vi "Drive_Initialize.vi"(11 "HW SETUP_WC Drive":T1={"Left Master"=3, "Invert Left Master"=FALSE, "Left Slave"=6, "Invert Left Slave"=FALSE, "Right Master"=12, "Invert Right Master"=FALSE, "Right Slave"=13, "Invert Right Slave"=FALSE, "Invert Left Encoder"=TRUE, "Invert Right Encoder"=FALSE}) -> (3 "RobotDriveDevRef Out":T2)   [LabVIEW 2017, in "WCDrive2018.lvlib"]
uses:
  WCDrive2018.lvlib
  <vilib>/Rock Robotics/WPI/RobotDrive/WPI_RobotDriveDevRef.ctl
  <vilib>/Rock Robotics/WPI/MotorControl/WPI_MotorControlDeviceRef.ctl
  <vilib>/Rock Robotics/WPI/MotorControl/WPI_MotorControlType.ctl
  <vilib>/Rock Robotics/SystemInterfaces/DIO/FPGA_DIOPWMChannel.ctl
  <vilib>/Rock Robotics/WPI/PWM/WPI_PWMDeadband.ctl
  <vilib>/Rock Robotics/SystemInterfaces/DIO/FPGA_DIOChannel.ctl
  ProtoType Code/Claw Testing/Systems/WCDrive2018/Cluster_WCDrive_SetupData.ctl
  System Drivers/Phoenix-LabVIEW/Motor Controller/Controls/CTRE_Phoenix_MotorControl_FeedbackDevice.ctl
  System Drivers/Phoenix-LabVIEW/Motor Controller/Controls/CTRE_Phoenix_MotorControl_NeutralMode.ctl
  <vilib>/Rock Robotics/WPI/RobotDrive/WPI_RobotDriveOpen4MotorWithExistingMotors.vi
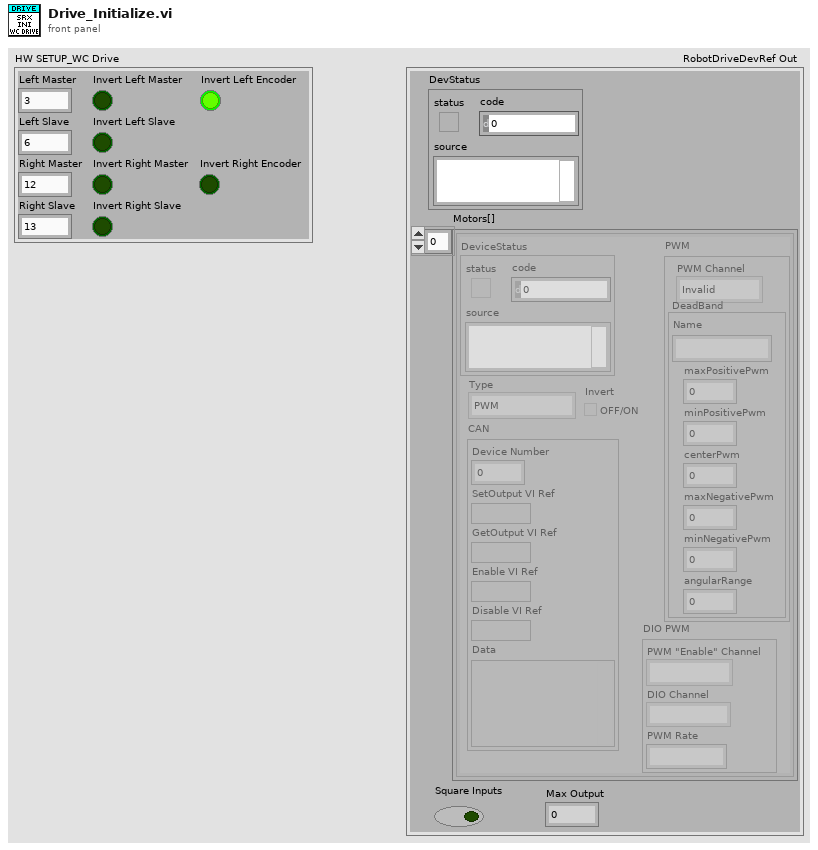
[diagram p1: front panel]
types:
  T1 = typedef "Cluster_WCDrive_SetupData.ctl" = cluster{"Left Master":u8, "Invert Left Master":bool, "Left Slave":u8, "Invert Left Slave":bool, "Right Master":u8, "Invert Right Master":bool, "Right Slave":u8, "Invert Right Slave":bool, "Invert Left Encoder":bool, "Invert Right Encoder":bool}
  T2 = typedef "WPI_RobotDriveDevRef.ctl" = cluster{"DevStatus":errorcluster, "Motors[]":T3[], "Square Inputs":bool, "Max Output":dbl}
  T3 = typedef "WPI_MotorControlDeviceRef.ctl" = cluster{"DeviceStatus":errorcluster, "Type":T4, "PWM":cluster{"PWM Channel":T5, "DeadBand":T6}, "CAN":cluster{"Device Number":u8, "SetOutput VI Ref":variant, "GetOutput VI Ref":variant, "Enable VI Ref":variant, "Disable VI Ref":variant, "Data":variant}, "Invert":bool, "DIO PWM":cluster{"PWM \"Enable\" Channel":T5, "DIOChannel":T7, "PWM Rate":dbl}}
  T4 = typedef "WPI_MotorControlType.ctl" = enum16{"PWM", "CAN", "DIO PWM"}
  T5 = typedef "FPGA_DIOPWMChannel.ctl" = enum8{"PWM 0", "PWM 1", "PWM 2", "PWM 3", "PWM 4", "PWM 5", "PWM 6", "PWM 7", "PWM 8", "PWM 9", "PWM MXP 0", "PWM MXP 1", "PWM MXP 2", "PWM MXP 3", "PWM MXP 4", "PWM MXP 5", "PWM MXP 6", "PWM MXP 7", "PWM MXP 8", "PWM MXP 9", "Invalid"}
  T6 = typedef "WPI_PWMDeadband.ctl" = cluster{"Name":string, "maxPositivePwm":i32, "minPositivePwm":i32, "centerPwm":i32, "maxNegativePwm":i32, "minNegativePwm":i32, "angularRange":u16}
  T7 = typedef "FPGA_DIOChannel.ctl" = enum8{"DIO 0", "DIO 1", "DIO 2", "DIO 3", "DIO 4", "DIO 5", "DIO 6", "DIO 7", "DIO 8", "DIO 9", "DIO MXP 0", "DIO MXP 1", "DIO MXP 2", "DIO MXP 3", "DIO MXP 4", "DIO MXP 5", "DIO MXP 6", "DIO MXP 7", "DIO MXP 8", "DIO MXP 9", "DIO MXP 10", "DIO MXP 11", "DIO MXP 12", "DIO MXP 13", "DIO MXP 14", "DIO MXP 15", "SPI Port CS1", "SPI Port CS2", "SPI Port CS3", "SPI Port MISO", "SPI Port MOSI", "Invalid"}
  T8 = typedef "CTRE_Phoenix_MotorControl_NeutralMode.ctl" = enum8{"EEPROMSetting", "Override to Coast", "Override to Brake"}
  T9 = typedef "CTRE_Phoenix_MotorControl_FeedbackDevice.ctl" = i8
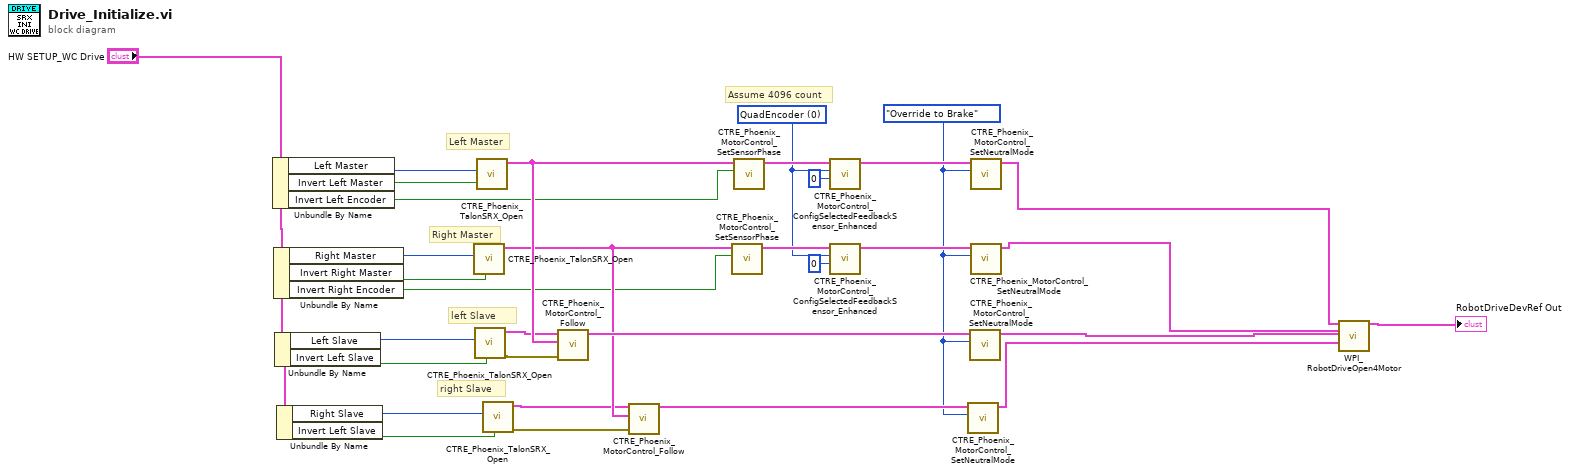
[diagram p0: block diagram]
diagram:
  w22 = CTRE_Phoenix_MotorControl_NeutralMode."Override to Brake" ("Motor Control Neutral Mode")
  w25 = T9 0 items=["None"=-1, "QuadEncoder"=0, "Analog"=2, "Tachometer"=4, "Pulse Width Encoded Position"=8, "Sensor Sum (S0 + S1)"=9, "Sensor Difference (D0 - D1)"=10, "Remote Source 0"=11, "Remote Source 1"=12, "Software Emulated"=15] ("Feedback Device")
  # "right Slave"
  # "Assume 4096 count"
  # "left Slave"
  # "Right Master"
  # "Left Master"
  n1 = Unbundle By Name("HW SETUP_WC Drive") -> ("Left Master"=w14:u8, "Invert Left Master"=w13:bool, "Invert Left Encoder"=w6:bool)
  n2 = Unbundle By Name("HW SETUP_WC Drive") -> ("Right Master"=w12:u8, "Invert Right Master"=w11:bool, "Invert Right Encoder"=w5:bool)
  n3 = Unbundle By Name("HW SETUP_WC Drive") -> ("Left Slave"=w10:u8, "Invert Left Slave"=w9:bool)
  n4 = Unbundle By Name("HW SETUP_WC Drive") -> ("Right Slave"=w8:u8, "Invert Left Slave"=w7:bool)
  n5 = call "CTRE_Phoenix_TalonSRX_Open.vi"("Invert"=w11, "Device Number"=w12) -> ("CAN Talon SRX Ref"=w29:T3)  [unwired: 8 in, 1 out]
  n6 = call "CTRE_Phoenix_TalonSRX_Open.vi"("Invert"=w9, "Device Number"=w10) -> ("error out"=w18:errorcluster, "CAN Talon SRX Ref"=w19:T3)  [unwired: 8 in]
  n7 = call "CTRE_Phoenix_TalonSRX_Open.vi"("Invert"=w13, "Device Number"=w14) -> ("CAN Talon SRX Ref"=w31:T3)  [unwired: 8 in, 1 out]
  n8 = call "CTRE_Phoenix_TalonSRX_Open.vi"("Invert"=w7, "Device Number"=w8) -> ("error out"=w16:errorcluster, "CAN Talon SRX Ref"=w17:T3)  [unwired: 8 in]
  n9 = call "CTRE_Phoenix_MotorControl_Follow.vi"("error in (no error)"=w18, "Master Controller to Follow"=w31, "PhoenixMotorControlDevRef"=w19) -> ("PhoenixMotorControlDevRef"=w30:T3)  [unwired: 7 in, 1 out]
  n10 = call "CTRE_Phoenix_MotorControl_Follow.vi"("error in (no error)"=w16, "Master Controller to Follow"=w29, "PhoenixMotorControlDevRef"=w17) -> ("PhoenixMotorControlDevRef"=w28:T3)  [unwired: 7 in, 1 out]
  n11 = call "CTRE_Phoenix_MotorControl_SetSensorPhase.vi"("PhaseSensor"=w5, "PhoenixMotorControlDevRef"=w29) -> ("PhoenixMotorControlDevRef"=w26:T3)  [unwired: 8 in, 1 out]
  n12 = call "CTRE_Phoenix_MotorControl_SetSensorPhase.vi"("PhaseSensor"=w6, "PhoenixMotorControlDevRef"=w31) -> ("PhoenixMotorControlDevRef"=w27:T3)  [unwired: 8 in, 1 out]
  n13 = call "CTRE_Phoenix_MotorControl_ConfigSelectedFeedbackSensor_Enhanced.vi"("PidLoopIdx"=0 ("pidLoopIdx"), "Feedback Device"=w25, "PhoenixMotorControlDevRef"=w27) -> ("PhoenixMotorControlDevRef Out"=w24:T3)  [unwired: 7 in, 1 out]
  n14 = call "CTRE_Phoenix_MotorControl_ConfigSelectedFeedbackSensor_Enhanced.vi"("PidLoopIdx"=0 ("pidLoopIdx"), "Feedback Device"=w25, "PhoenixMotorControlDevRef"=w26) -> ("PhoenixMotorControlDevRef Out"=w23:T3)  [unwired: 7 in, 1 out]
  n15 = call "CTRE_Phoenix_MotorControl_SetNeutralMode.vi"("Motor Control Neutral Mode"=w22, "PhoenixMotorControlDevRef"=w28) -> ("PhoenixMotorControlDevRef Out"=w1:T3)  [unwired: 8 in, 1 out]
  n16 = call "CTRE_Phoenix_MotorControl_SetNeutralMode.vi"("Motor Control Neutral Mode"=w22, "PhoenixMotorControlDevRef"=w30) -> ("PhoenixMotorControlDevRef Out"=w2:T3)  [unwired: 8 in, 1 out]
  n17 = call "CTRE_Phoenix_MotorControl_SetNeutralMode.vi"("Motor Control Neutral Mode"=w22, "PhoenixMotorControlDevRef"=w24) -> ("PhoenixMotorControlDevRef Out"=w4:T3)  [unwired: 8 in, 1 out]
  n18 = call "CTRE_Phoenix_MotorControl_SetNeutralMode.vi"("Motor Control Neutral Mode"=w22, "PhoenixMotorControlDevRef"=w23) -> ("PhoenixMotorControlDevRef Out"=w3:T3)  [unwired: 8 in, 1 out]
  n19 = call-poly <vilib>:"WPI_RobotDriveOpen4Motor.vi"("Rear Left Motor Dev Ref"=w4, "Rear Right Motor Dev Ref"=w3, "Front Left Motor Dev Ref"=w2, "Front Right Motor Dev Ref"=w1) -> ("RobotDriveDevRef"=→"RobotDriveDevRef Out":T2)  [unwired: 10 in, 1 out]
